vi "buffer array 1D.vi"(0 "Array":dbl[](array[numeric]), 1 "History length":i32, 2 "Log":T1=enum."TimeStamp", 10 "Start channel":i32) -> ()   [LabVIEW 2018]
uses:
  history_array_type.ctl
  CAEN globals.vi
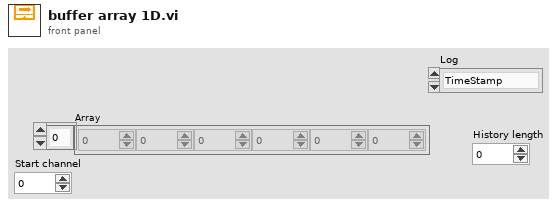
[diagram p1: front panel]
types:
  T1 = typedef "history_array_type.ctl" = enum16{"Vmon", "Vset", "Imon", "Iset", "TimeStamp"}
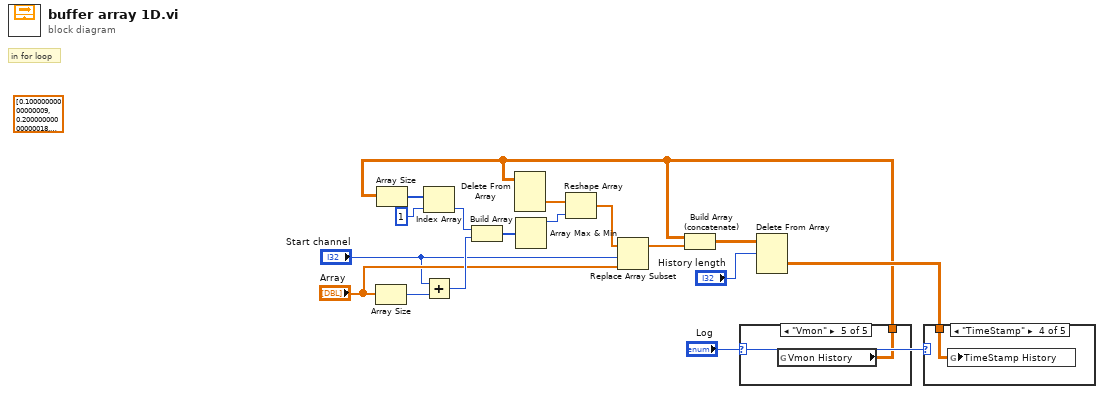
[diagram p0: block diagram]
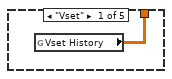
[diagram p2: hidden frame]
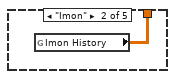
[diagram p3: hidden frame]
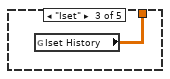
[diagram p4: hidden frame]
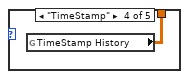
[diagram p5: hidden frame]
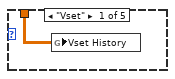
[diagram p6: hidden frame]
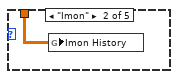
[diagram p7: hidden frame]
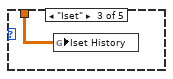
[diagram p8: hidden frame]
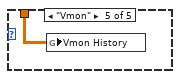
[diagram p9: hidden frame]
diagram:
  (unwired) dbl[][] [[0.10000000000000009, 0.20000000000000018, 1.2999999999999998], [1.1, 1.2, 1.3], [2.1, 2.2, 2.3], [3.1, 3.2, 3.3], [4.1, 4.2, 4.3], [5.1, 5.2, 5.3]] ("Test")
  # "in for loop"
  n1 = Array Size(array="Array") -> (size(s)=w17:i32)
  n2 = Add(x="Start channel", y=w17) -> (x+y=w15:i32)
  n3 = case shown="\"Vmon\"" "Log" {
    tunnel: [w18 w19 w20 w21 w22] -> w1
    frame "Vset" {
      n4 = global read "CAEN globals.vi" "Vset History"() -> (w18:dbl[][])
    }
    frame "Imon" {
      n5 = global read "CAEN globals.vi" "Imon History"() -> (w19:dbl[][])
    }
    frame "Iset" {
      n6 = global read "CAEN globals.vi" "Iset History"() -> (w20:dbl[][])
    }
    frame "TimeStamp" {
      n7 = global read "CAEN globals.vi" "TimeStamp History"() -> (w21:dbl[][])
    }
    frame "Vmon" {
      n8 = global read "CAEN globals.vi" "Vmon History"() -> (w22:dbl[][])
    }
  }
  n9 = Array Size(array=w1) -> (size(s)=w16:i32[])
  n10 = Index Array(array=w16, index=1) -> (element=w10:i32)
  n11 = Build Array(w10, w15) -> (w14:i32[])
  n12 = Delete From Array(array=w1) -> (deleted portion=w6:dbl[])  [unwired: 3 in, 1 out]
  n13 = Array Max & Min(array=w14) -> (max value=w5:i32)  [unwired: 3 out]
  n14 = Reshape Array(w6, w5) -> (w4:dbl[])
  n15 = Replace Array Subset(array=w4, new element="Array", index="Start channel") -> (w7:dbl[])
  n16 = Build Array (concatenate)(w1, w7) -> (w13:dbl[][])
  n17 = Delete From Array(array=w13, length="History length") -> (deleted portion=w3:dbl[][])  [unwired: 2 in, 1 out]
  n18 = case shown="\"TimeStamp\"" "Log" {
    tunnel: w3 -> [w23 w24 w25 w26 w27]
    frame "Vset" {
      n19 = global write "CAEN globals.vi" "Vset History"(w23) -> ()
    }
    frame "Imon" {
      n20 = global write "CAEN globals.vi" "Imon History"(w24) -> ()
    }
    frame "Iset" {
      n21 = global write "CAEN globals.vi" "Iset History"(w25) -> ()
    }
    frame "TimeStamp" {
      n22 = global write "CAEN globals.vi" "TimeStamp History"(w26) -> ()
    }
    frame "Vmon" {
      n23 = global write "CAEN globals.vi" "Vmon History"(w27) -> ()
    }
  }
